vi "ExecuteControl.vi"(11 "StateParams":T1) -> (3 "RobotControl":cluster{"VlProfile":i16[], "VrProfile":i16[]})   [LabVIEW 2011]
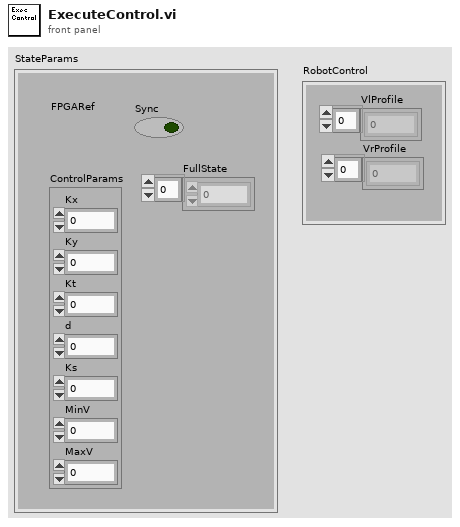
[diagram p1: front panel]
types:
  T1 = cluster{"FPGARef":refnum<k20>, "Sync":bool, "ControlParams":cluster{"Kx":dbl, "Ky":dbl, "Kt":dbl, "d":dbl, "Ks":dbl, "MinV":i16, "MaxV":i16}, "FullState":dbl[]}
  T2 = cluster{"Kx":dbl, "Ky":dbl, "Kt":dbl, "d":dbl, "Ks":dbl, "MinV":i16, "MaxV":i16}
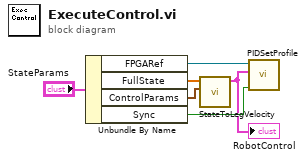
[diagram p0: block diagram]
diagram:
  n1 = Unbundle By Name("StateParams") -> ("FPGARef"=w5:refnum<k20>, "FullState"=w4:dbl[], "ControlParams"=w3:T2, "Sync"=w2:bool)
  n2 = call "StateToLegVelocity.vi"("ControlParams"=w3, "State"=w4) -> ("RobotControl"=w1:cluster{"VlProfile":i16[], "VrProfile":i16[]})  [unwired: 8 in]
  "RobotControl" <- w1
  n3 = call "PIDSetProfile.vi"("Refnum in"=w5, "RobotControl"=w1, "Sync"=w2) -> ()  [unwired: 6 in, 1 out]
